vi "AB_RW_Project_Deploy_EXE_Info.vi"(7 "action":T1, 8 "error in (no error)":errorcluster, 10 "info in":T2, 11 "Object In":T3) -> (0 "error out":errorcluster, 2 "info out":T2, 3 "Object Out":T3)   [LabVIEW 2020]
uses:
  <vilib>/AppBuilder/RW_Project/AB_RW_Project_PropBag_Action.ctl
  <vilib>/AppBuilder/RW_Project/AB_RW_Project_Deploy_EXE_Data.ctl
  <resource>/Framework/Providers/API/ItemRef.ctl
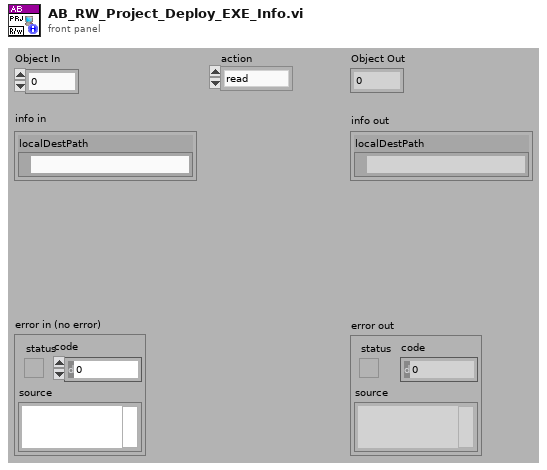
[diagram p1: front panel]
types:
  T1 = typedef "AB_RW_Project_PropBag_Action.ctl" = enum16{"read", "write", "clear", "readPrevious", "writePrevious", "clearPrevious"}
  T2 = typedef "AB_RW_Project_Deploy_EXE_Data.ctl" = cluster{"localDestPath":path}
  T3 = typedef "ItemRef.ctl" = u64
  T4 = typedef "AB_Relative_Path_Type.ctl" = enum16{"<none>", "relativeToCommon", "relativeToAppDir", "relativeToProject"}
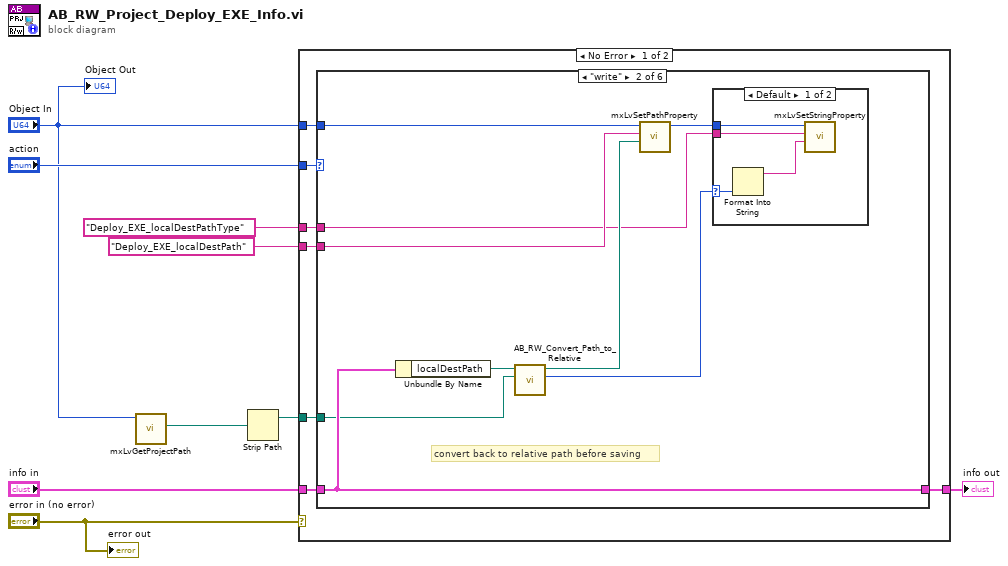
[diagram p0: block diagram]
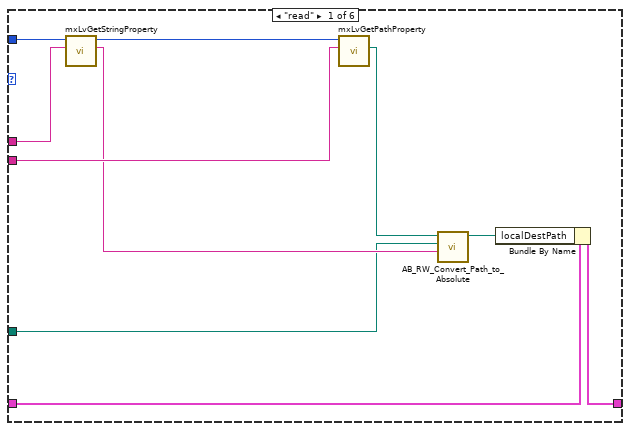
[diagram p2: hidden frame]
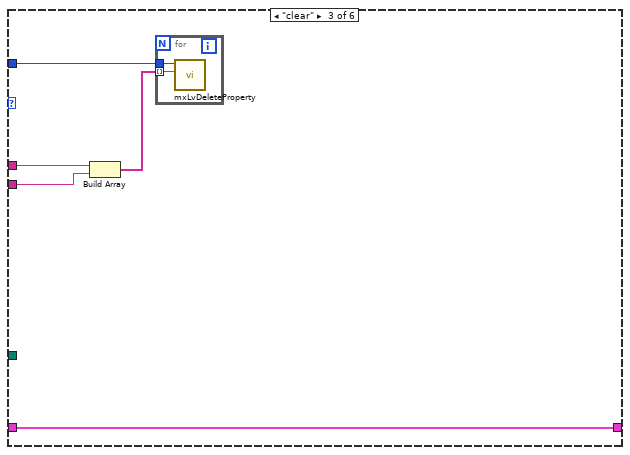
[diagram p4: hidden frame]
diagram:
  n1 = call <resource>:"mxLvGetProjectPath.vi"("Item"="Object In") -> ("Project Path"=w1:path)  [unwired: 8 in, 2 out]
  n2 = Strip Path(path=w1) -> (stripped path=w3:path)  [unwired: 1 out]
  n3 = case shown="No Error" "error in (no error)" {
    tunnel: "Object In" -> [w15 _]
    tunnel: [w16 _] -> w8
    tunnel: "info in" -> [w14 _]
    tunnel: "action" -> [w13 _]
    tunnel: "Deploy_EXE_localDestPath" ("Tag") -> [w12 _]
    tunnel: "Deploy_EXE_localDestPathType" ("Tag") -> [w11 _]
    tunnel: w3 -> [w10 _]
    frame No Error {
      n4 = case shown="\"write\"" w13 {
        tunnel: [w26 w35 w44 w47 w48 w49] -> w16
        tunnel: w15 -> [w23 w28 w43 _ _ _]
        tunnel: w14 -> [w25 w35 w44 w47 w48 w49]
        tunnel: w12 -> [w24 w34 w41 _ _ _]
        tunnel: w11 -> [w21 w27 w40 _ _ _]
        tunnel: w10 -> [w18 w31 _ _ _ _]
        frame "read" {
          n5 = call <resource>:"mxLvGetStringProperty.vi"("Tag"=w21, "Item"=w23) -> ("Value"=w20:string, "Item"=w22:T3)  [unwired: 7 in, 1 out]
          n6 = call <resource>:"mxLvGetPathProperty.vi"("Tag"=w24, "Item"=w22) -> ("Path"=w19:path)  [unwired: 7 in, 2 out]
          n7 = call <vilib>:"AB_RW_Convert_Path_to_Absolute.vi"("relativeType"=w20, "commonPath"=w18, "relativePath"=w19) -> ("absolute path"=w17:path)  [unwired: 7 in, 1 out]
          n8 = Bundle By Name(cluster=w25, "localDestPath"=w17) -> (w26:T2)
        }
        frame "write" {
          # "convert back to relative path before saving"
          n9 = Unbundle By Name(w35) -> ("localDestPath"=w33:path)
          n10 = call <vilib>:"AB_RW_Convert_Path_to_Relative.vi"("commonPath"=w31, "absolutePath"=w33) -> ("relativeType"=w30:T4, "newPath"=w32:path)  [unwired: 7 in, 1 out]
          n11 = call <resource>:"mxLvSetPathProperty.vi"("Path"=w32, "Tag"=w34, "Item"=w28) -> ("Item"=w29:T3)  [unwired: 7 in, 1 out]
          n12 = case shown="Default" w30 {
            selector: w30 -> [w38 _]
            tunnel: w29 -> [w39 _]
            tunnel: w27 -> [w36 _]
            frame Default {
              n13 = Format Into String(w38) -> (resulting string=w37:string)  [unwired: 3 in, 1 out]
              n14 = call <resource>:"mxLvSetStringProperty.vi"("Value (\"\")"=w37, "Tag"=w36, "Item"=w39) -> ()  [unwired: 7 in, 2 out]
            }
            frame "relativeToCommon" {
            }
          }
        }
        frame "clear" {
          n15 = Build Array(w40, w41) -> (w42:string[])
          n16 = for {
            tunnel: w43 -> [w46]
            tunnel: w42 -> [w45] mode=indexing
            n17 = call <resource>:"mxLvDeleteProperty.vi"("Tag"=w45, "Item"=w46) -> ()  [unwired: 8 in, 2 out]
          }
        }
        frame "readPrevious" {
        }
        frame "writePrevious" {
        }
        frame "clearPrevious" {
        }
      }
    }
    frame Error {
    }
  }
  "info out" <- w8
  "Object Out" <- "Object In"
  "error out" <- "error in (no error)"
